vi "Align Needle Dialog.vi"(7 "Console Log in":refnum<class "Console Log.lvclass">, 8 "error in":errorcluster, 11 "Potting Procedure in":refnum<class "Potting Procedure.lvclass">) -> (0 "error out":errorcluster, 2 "Canceled":bool, 3 "Potting Procedure out":refnum<class "Potting Procedure.lvclass">, 5 "Console Log out":refnum<class "Console Log.lvclass">)   [LabVIEW 2017]
uses:
  Procedure Classes/Potting Procedure/Potting Procedure.lvclass
  Shared Components/Gantry Class/Gantry Class.lvclass
  Shared Components/Vec3d Class/Vec3d Class.lvclass
  Shared Components/WorkTable Class/WorkTable Class.lvclass
  Shared Components/Config Manager Class/Type Definitions/Named Position.ctl
  Shared Components/Config Manager Class/Type Definitions/Camera Enum.ctl
  Application Utilities/Console Log/Console Log.lvclass
panel:
  out "Offset(mm)":cluster{"X":dbl, "Y":dbl, "Z":dbl}
  in  "Camera Selection":T1(radio)
  out "preview":T2(plugin-control)
  in  "OK Button":bool
  in  "Cancel Button":bool
  # "Use the MPG  hand control to\nmove the needle tip to the center\nof the image in both X and Y"
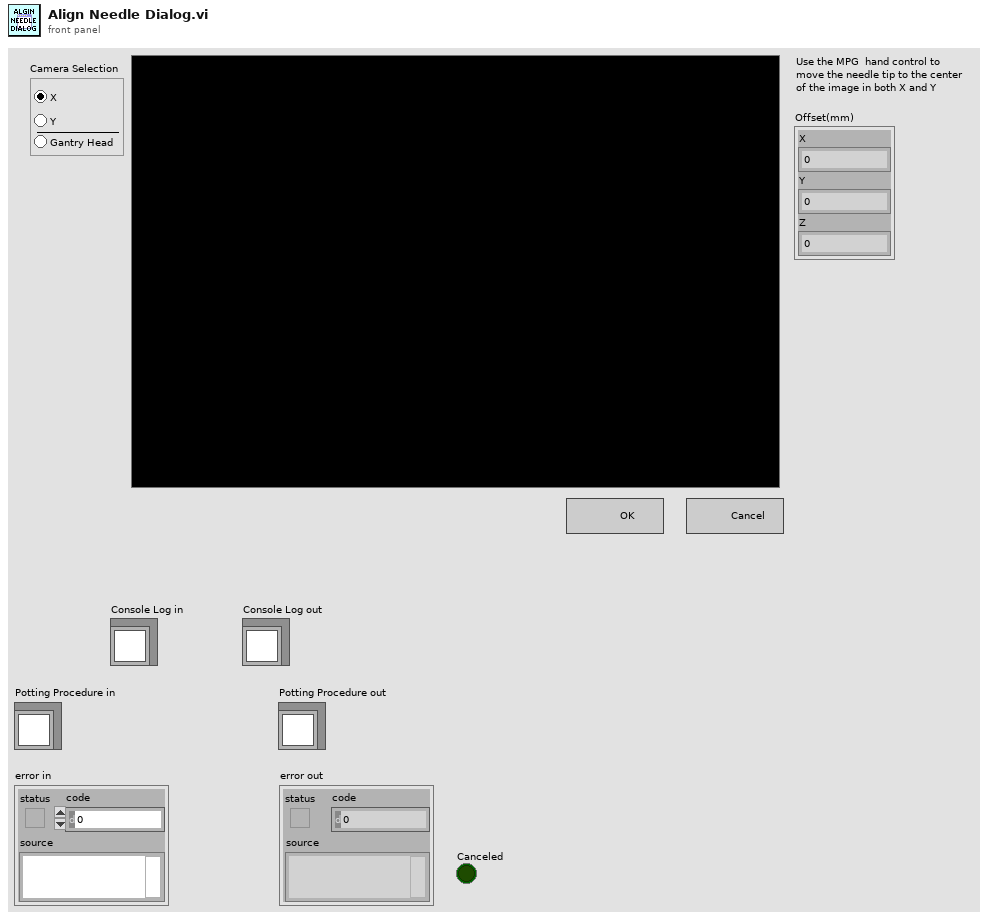
[diagram p1: front panel]
types:
  T1 = enum32{"Radio Selection 1", "Radio Selection 2", "Radio Selection 3"}
  T2 = typedef "IMAQ Image.ctl" = refnum<image>
  T3 = typedef "Named Position.ctl" = enum16{"home", "module_chuck_0", "module_chuck_1", "module_chuck_2", "module_chuck_3", "module_chuck_4", "glue_reservoir_chuck", "stamp_tool_chuck", "weight_tool_chuck", "needle_calibration", "needle_calibration_camera", "tool_rack_pos_0_in", "tool_rack_pos_0_out", "tool_rack_pos_1_in", "tool_rack_pos_1_out", "tool_rack_pos_2_in", "tool_rack_pos_2_out", "front_load_position", "grabber_start_pos", "between_chuck_0_and_1", "between_chuck_2_and_3"}
  T4 = enum8{"Enabled", "Disabled", "Disabled and Grayed Out"}
  T5 = typedef "Camera Enum.ctl" = enum16{"GANTRY HEAD", "NEEDLE CALIBRATION X", "NEEDLE CALIBRATION Y"}
  T6 = typedef "Physical Image.ctl" = cluster{"Image Position":refnum<class "Vec3d Class.lvclass">, "Image Reference":T2, "Field of View":cluster{"x(mm)":dbl, "y(mm)":dbl}}
  T7 = typedef "Worktable_Syringe.ctl" = cluster{"Syringe Holder":enum16{"Empty", "Populated", "Calibrated"}, "Mixing Time":timestamp, "Tip Offset":refnum<class "Vec3d Class.lvclass">}
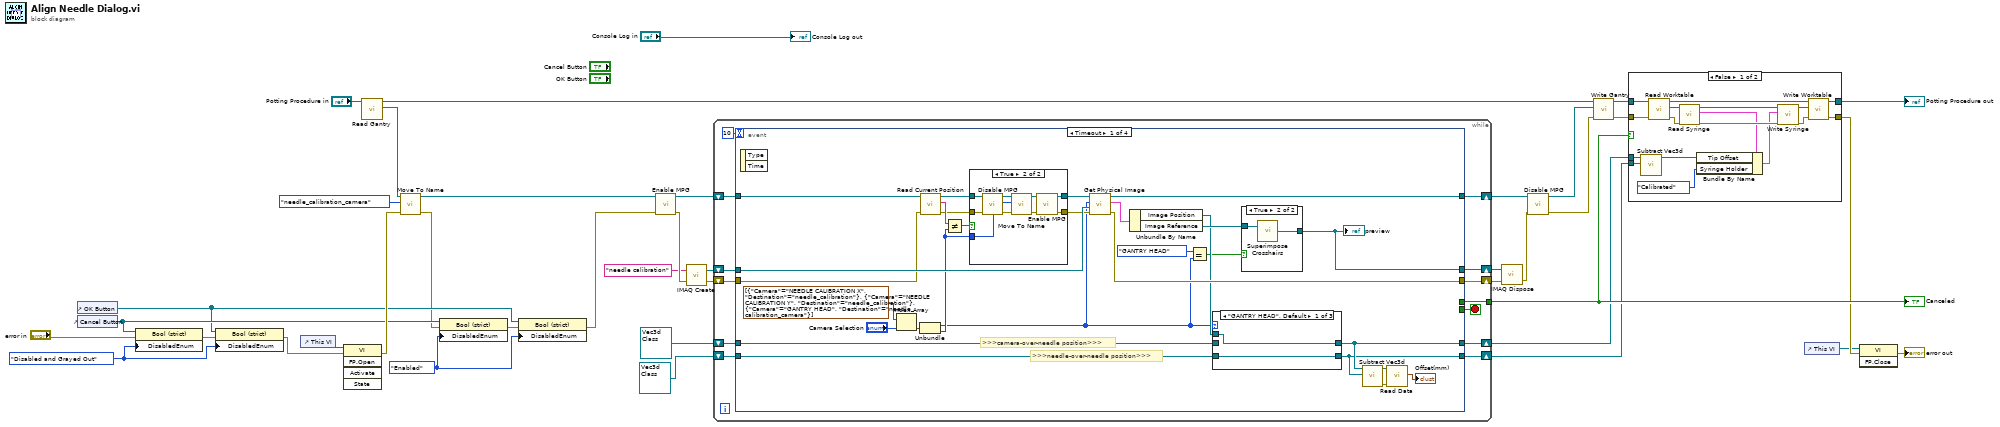
[diagram p0: block diagram]
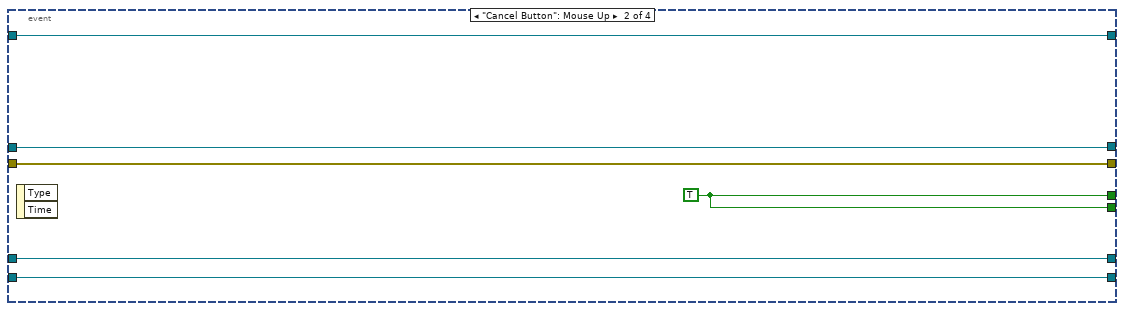
[diagram p7: hidden frame]
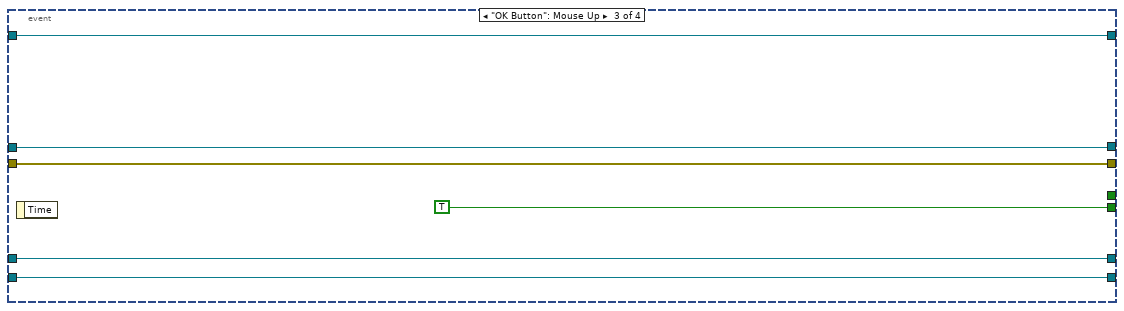
[diagram p8: hidden frame]
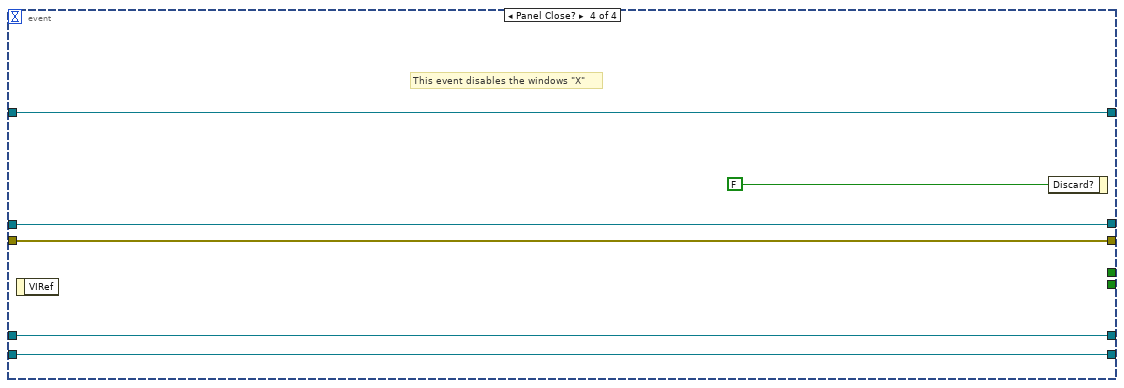
[diagram p9: hidden frame]
diagram:
  w16 = T4."Enabled" ("Disabled")
  w17 = T4."Disabled and Grayed Out" ("Disabled")
  n1 = control-ref of="OK Button"() -> (w18:refnum<vi>)
  n2 = control-ref of="Cancel Button"() -> (w19:refnum<vi>)
  n3 = property class="Bool (strict)"(reference=w19, error in="error in", "DisabledEnum"=w17) -> (error out=w21:errorcluster)  [unwired: 1 out]
  n4 = property class="Bool (strict)"(reference=w18, error in=w21, "DisabledEnum"=w17) -> (error out=w15:errorcluster)  [unwired: 1 out]
  n5 = control-ref of="This VI"() -> (w40:refnum<vi>)
  n6 = invoke class="VI" method="FP.Open"(reference=w40, error in=w15) -> (error out=w36:errorcluster)  [unwired: 3 in, 4 out]
  n7 = call-dynamic "Read Gantry.vi"("Potting Procedure in"="Potting Procedure in") -> ("Gantry"=w37:refnum<class "Gantry Class.lvclass">, "Potting Procedure out"=w25:refnum<class "Potting Procedure.lvclass">)  [unwired: 8 in, 1 out]
  n8 = call-dynamic "Move To Name.vi"("error in"=w36, "Destination"=Named_Position."needle_calibration_camera", "Gantry in"=w37) -> ("error out"=w13:errorcluster, "Gantry out"=w10:refnum<class "Gantry Class.lvclass">)  [unwired: 7 in]
  n9 = property class="Bool (strict)"(reference=w19, error in=w13, "DisabledEnum"=w16) -> (error out=w20:errorcluster)  [unwired: 1 out]
  n10 = property class="Bool (strict)"(reference=w18, error in=w20, "DisabledEnum"=w16) -> (error out=w9:errorcluster)  [unwired: 1 out]
  n11 = call-dynamic "Enable MPG.vi"("error in"=w9, "Gantry in"=w10) -> ("error out"=w33:errorcluster, "Gantry out"=w35:refnum<class "Gantry Class.lvclass">)  [unwired: 8 in]
  n12 = call "IMAQ Create"("Image Name"="needle calibration", "error in (no error)"=w33) -> ("New Image"=w30:T2, "error out"=w31:errorcluster)  [unwired: 3 in]
  n13 = while {
    tunnel: [w49] -> w26
    shift-right: [w47] -> w34
    shift-left: w35 -> [w48]
    shift-right: [w51] -> w29
    shift-left: w31 -> [w50]
    shift-right: [w45] -> w28
    shift-left: w30 -> [w46]
    shift-right: [w42] -> w4
    shift-left: refnum<class "Vec3d Class.lvclass"> refnum ("Vec3d Class.lvclass") -> [w44]
    shift-right: [w41] -> w3
    shift-left: refnum<class "Vec3d Class.lvclass"> refnum ("Vec3d Class.lvclass") -> [w43]
    stop <- w52 stop-if-true
    n14 = event shown="[0] Timeout" {
      selector: _ -> [_ _ _ _]
      dyn-events: _ -> [_ _ _ _]
      timeout: 10 -> [_ _ _ _]
      tunnel: [_ w107 TRUE _] -> w52
      tunnel: [w76 w108 w114 w119] -> w51
      tunnel: w50 -> [w67 w108 w114 w119]
      tunnel: [_ w107 _ _] -> w49
      tunnel: w48 -> [w73 w106 w112 w118]
      tunnel: [w80 w106 w112 w118] -> w47
      tunnel: w46 -> [w77 w105 w111 w117]
      tunnel: [w75 w105 w111 w117] -> w45
      tunnel: w44 -> [w63 w104 w110 w116]
      tunnel: w43 -> [w62 w103 w109 w115]
      tunnel: [w61 w104 w110 w116] -> w42
      tunnel: [w60 w103 w109 w115] -> w41
      event Timeout {
        # ">>>needle-over-needle position>>>"
        # ">>>camera-over-needle position>>>"
        n15 = event-data() -> ()  [unwired: 1 in, 2 out]
        n16 = Index Array(array=cluster{"Camera":T5, "Destination":T3}[] [{"Camera"=enum."NEEDLE CALIBRATION X", "Destination"=enum."needle_calibration"}, {"Camera"=enum."NEEDLE CALIBRATION Y", "Destination"=enum."needle_calibration"}, {"Camera"=enum."GANTRY HEAD", "Destination"=enum."needle_calibration_camera"}], index="Camera Selection") -> (element=w74:cluster{"Camera":T5, "Destination":T3})
        n17 = Unbundle(w74) -> ("Camera"=w56:T5, "Destination"=w70:T3)
        n18 = call-dynamic "Read Current Position.vi"("error in"=w67, "Gantry in"=w73) -> ("error out"=w68:errorcluster, "Current Position"=w72:string, "Gantry out"=w71:refnum<class "Gantry Class.lvclass">)  [unwired: 7 in]
        n19 = Not Equal?(x=w72, y=w70) -> (x != y?=w69:bool)
        n20 = case shown="True" w69 {
          tunnel: w71 -> [w93 w102]
          tunnel: w70 -> [_ w96]
          tunnel: w68 -> [w92 w99]
          tunnel: [w93 w95] -> w66
          tunnel: [w92 w94] -> w65
          frame False {
          }
          frame True {
            n21 = call-dynamic "Disable MPG.vi"("error in"=w99, "Gantry in"=w102) -> ("error out"=w100:errorcluster, "Gantry out"=w101:refnum<class "Gantry Class.lvclass">)  [unwired: 8 in]
            n22 = call-dynamic "Move To Name.vi"("error in"=w100, "Destination"=w96, "Gantry in"=w101) -> ("error out"=w97:errorcluster, "Gantry out"=w98:refnum<class "Gantry Class.lvclass">)  [unwired: 7 in]
            n23 = call-dynamic "Enable MPG.vi"("error in"=w97, "Gantry in"=w98) -> ("error out"=w94:errorcluster, "Gantry out"=w95:refnum<class "Gantry Class.lvclass">)  [unwired: 8 in]
          }
        }
        n24 = call-dynamic "Get Physical Image.vi"("error in"=w65, "Image In"=w77, "Camera Name"=w56, "Gantry in"=w66) -> ("error out"=w76:errorcluster, "Physical Image"=w79:T6, "Gantry out"=w80:refnum<class "Gantry Class.lvclass">)  [unwired: 5 in]
        n25 = Unbundle By Name(w79) -> ("Image Position"=w64:refnum<class "Vec3d Class.lvclass">, "Image Reference"=w78:T2)
        n26 = Equal?(x=Camera_Enum."GANTRY HEAD", y=w56) -> (x = y?=w54:bool)
        n27 = case shown="\"GANTRY HEAD\", Default" w56 {
          tunnel: w64 -> [w86 w88 w91]
          tunnel: w63 -> [_ w89 w90]
          tunnel: w62 -> [w87 _ _]
          tunnel: [w87 w88 w91] -> w60
          tunnel: [w86 w89 w90] -> w61
          frame "GANTRY HEAD", Default {
          }
          frame "NEEDLE CALIBRATION X" {
          }
          frame "NEEDLE CALIBRATION Y" {
          }
        }
        n28 = case shown="True" w54 {
          tunnel: w78 -> [w83 w85]
          tunnel: [w83 w84] -> w75
          frame False {
          }
          frame True {
            n29 = call "Superimpose Crosshairs.vi"("Refnum in"=w85) -> ("Refnum out"=w84:T2)  [unwired: 1 in]
          }
        }
        "preview" <- w75
        n30 = call "Subtract Vec3d.vi"("Vec3d in 2"=w60, "Vec3d in 1"=w61) -> ("error out"=w59:errorcluster, "Vec3d Class out"=w58:refnum<class "Vec3d Class.lvclass">)  [unwired: 8 in]
        n31 = call-dynamic "Read Data.vi"("error in (no error)"=w59, "Vec3d Class in"=w58) -> ("Data"=→"Offset(mm)":cluster{"X":dbl, "Y":dbl, "Z":dbl})  [unwired: 7 in, 2 out]
      }
      event "Cancel Button": Mouse Up {
        w107 = TRUE
        n32 = event-data() -> ()  [unwired: 1 in, 2 out]
      }
      event "OK Button": Mouse Up {
        n33 = event-data() -> ()  [unwired: 1 in, 1 out]
      }
      event Panel Close? {
        # "This event disables the windows \"X\""
        n34 = event-data() -> ()  [unwired: 1 in, 1 out]
        n35 = event-data("Discard?"=FALSE) -> ()  [unwired: 1 in, 1 out]
      }
    }
  }
  "Canceled" <- w26
  n36 = call "IMAQ Dispose"("Image"=w28, "error in (no error)"=w29) -> ("error out"=w27:errorcluster)  [unwired: 4 in]
  n37 = call-dynamic "Disable MPG.vi"("error in"=w27, "Gantry in"=w34) -> ("error out"=w2:errorcluster, "Gantry out"=w5:refnum<class "Gantry Class.lvclass">)  [unwired: 8 in]
  n38 = call-dynamic "Write Gantry.vi"("error in (no error)"=w2, "Gantry"=w5, "Potting Procedure in"=w25) -> ("error out"=w1:errorcluster, "Potting Procedure out"=w24:refnum<class "Potting Procedure.lvclass">)  [unwired: 7 in]
  n39 = case shown="False" w26 {
    tunnel: w24 -> [w135 w139]
    tunnel: [w132 w139] -> w23
    tunnel: [w130 w138] -> w22
    tunnel: w4 -> [w126 _]
    tunnel: w3 -> [w125 _]
    tunnel: w1 -> [w123 w138]
    frame False {
      n40 = call "Subtract Vec3d.vi"("Vec3d in 2"=w125, "Vec3d in 1"=w126) -> ("Vec3d Class out"=w124:refnum<class "Vec3d Class.lvclass">)  [unwired: 8 in, 1 out]
      n41 = call-dynamic "Read Worktable.vi"("error in"=w123, "Potting Procedure in"=w135) -> ("error out"=w121:errorcluster, "WorkTable out"=w122:refnum<class "WorkTable Class.lvclass">, "Potting Procedure out"=w133:refnum<class "Potting Procedure.lvclass">)  [unwired: 7 in]
      n42 = call "Read Syringe.vi"("error in"=w121, "WorkTable in"=w122) -> ("error out"=w136:errorcluster, "Syringe"=w128:T7, "WorkTable out"=w137:refnum<class "WorkTable Class.lvclass">)  [unwired: 7 in]
      n43 = Bundle By Name(cluster=w128, "Tip Offset"=w124, "Syringe Holder"=enum16{"Empty", "Populated", "Calibrated"}."Calibrated") -> (w127:T7)
      n44 = call-dynamic "Write Syringe.vi"("error in (no error)"=w136, "Syringe"=w127, "WorkTable Class in"=w137) -> ("error out"=w131:errorcluster, "WorkTable Class out"=w134:refnum<class "WorkTable Class.lvclass">)  [unwired: 7 in]
      n45 = call-dynamic "Write Worktable.vi"("error in"=w131, "WorkTable in"=w134, "Potting Procedure in"=w133) -> ("error out"=w130:errorcluster, "Potting Procedure out"=w132:refnum<class "Potting Procedure.lvclass">)  [unwired: 7 in]
    }
    frame True {
    }
  }
  "Potting Procedure out" <- w23
  n46 = control-ref of="This VI"() -> (w8:refnum<vi>)
  n47 = invoke class="VI" method="FP.Close"(reference=w8, error in=w22) -> (error out=→"error out":errorcluster)  [unwired: 1 in, 2 out]
  "Console Log out" <- "Console Log in"
